vi "fake_read_constants.vi"(1 "line counter":u16, 3 "y resolution (nr. of lines)":u16) -> (0 "input cluster":T1)   [LabVIEW 2010]
uses:
  common_typedefs/channels_cluster.ctl
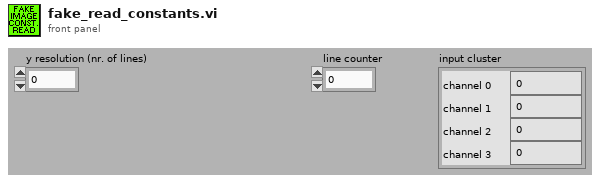
[diagram p1: front panel]
types:
  T1 = typedef "channels_cluster.ctl" = cluster{"channel 0":u32, "channel 1":u32, "channel 2":u32, "channel 3":u32}
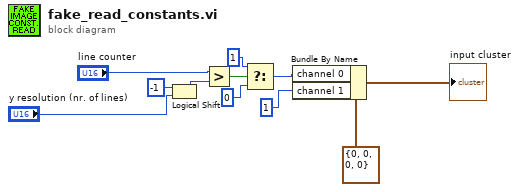
[diagram p0: block diagram]
diagram:
  n1 = Logical Shift(y=i16 -1 ("n"), x="y resolution (nr. of lines)") -> (x << y=w3:u16)
  n2 = Greater?(x="line counter", y=w3) -> (0:w1:bool)
  n3 = Select(t=u16 1 ("y"), s=w1, f=u16 0) -> (s? t:f=w9:u16)
  n4 = Bundle By Name(cluster=T1 {"channel 0"=0, "channel 1"=0, "channel 2"=0, "channel 3"=0} ("input cluster"), "channel 0"=w9, "channel 1"=u32 1) -> (→"input cluster":T1)
